vi "_memcpy.vi"(0 "MDPtr DVR":refnum<data-value>, 1 "Copy Count":i32, 5 "error in (no error)":errorcluster, 7 "Memory":string, 9 "String Attribute":string, 12 "Data Type":T1) -> (4 "MDPtr DVR(dup)":refnum<data-value>, 6 "error out":errorcluster)   [LabVIEW 2017, in "MDPtr.lvlib"]
uses:
  MDPtr.lvlib
  MDPtr TypeDef/MDPtr DataFrame-Memory.ctl
  MDPtr TypeDef/MDPtr DataFrame-Common.ctl
  <vilib>/Utility/Data Type/Type Definitions/Data Type.ctl
  _MDPtr Build Error Cluster.vi
  <vilib>/Utility/Data Type/NI_Data Type.lvlib
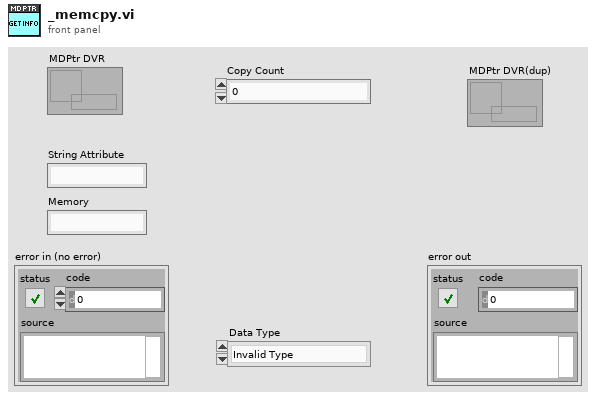
[diagram p1: front panel]
types:
  T1 = typedef "NI_Data Type.lvlib/Data Type.ctl" = enum8{"Invalid Type", "Void", "I8", "I16", "I32", "I64", "U8", "U16", "U32", "U64", "Single Float", "Double Float", "Extended Float", "Single Complex", "Double Complex", "Extended Complex", "Enum U8", "Enum U16", "Enum U32", "Enum U64", "Single Float With Unit", "Double Float With Unit", "Extended Float With Unit", "Single Complex with Unit", "Double Complex with Unit", "Extended Complex with Unit", "Boolean", "String", "Path", "Picture", "Tag", "Array", "Cluster", "Variant", "LV Variant", "Waveform", "Timestamp", "Digital Waveform", "Digital Data", "ExpressData", "Refnum", "External Data", "VI", "Poly VI", "LabVIEW Class Instance", "Fixed Point"}
  T2 = typedef "MDPtr.lvlib/MDPtr DataFrame-Memory.ctl" = cluster{"Common":T3, "DVR":refnum<data-value>}
  T3 = typedef "MDPtr.lvlib/MDPtr DataFrame-Common.ctl" = cluster{"Data Type":T1, "Copy Count":i32, "String Attribute":string, "Cache Length":i32, "Data Length":i32}
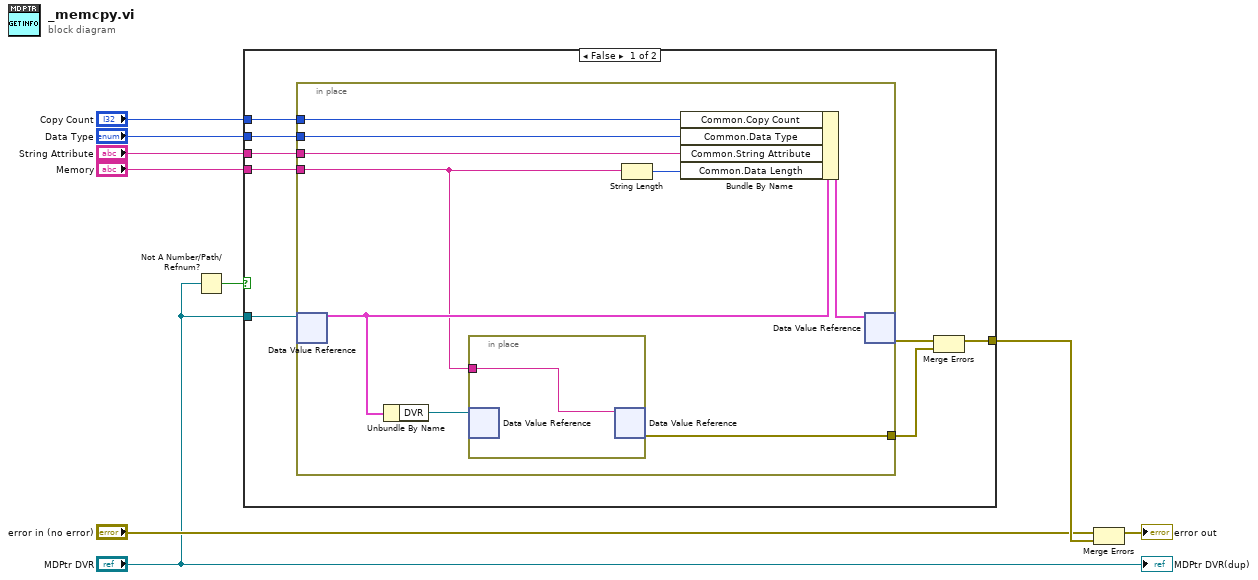
[diagram p0: block diagram]
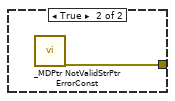
[diagram p2: hidden frame]
diagram:
  n1 = Not A Number/Path/Refnum?(number/path/refnum="MDPtr DVR") -> (NaN/Path/Refnum?=w5:bool)
  n2 = case shown="False" w5 {
    tunnel: [w11 w28] -> w9
    tunnel: "MDPtr DVR" -> [w16 _]
    tunnel: "Copy Count" -> [w15 _]
    tunnel: "Data Type" -> [w14 _]
    tunnel: "String Attribute" -> [w13 _]
    tunnel: "Memory" -> [w12 _]
    frame False {
      n3 = in-place {
        in-place-border: w15 -> [w25]
        in-place-border: w14 -> [w24]
        in-place-border: w13 -> [w23]
        in-place-border: w12 -> [w18]
        in-place-border: [w20] -> w10
        n4 = in-place-dvr #1(w16) -> (w22:T2)  [unwired: 1 out]
        n5 = Unbundle By Name(w22) -> ("DVR"=w21:refnum<data-value>)
        n6 = in-place {
          in-place-border: w18 -> [w27]
          n7 = in-place-dvr #2(w21) -> ()  [unwired: 2 out]
          n8 = in-place-dvr #2(w27) -> (w20:errorcluster)  [unwired: 1 out]
        }
        n9 = String Length(string=w18) -> (length=w19:i32)
        n10 = Bundle By Name(cluster=w22, "Common.Copy Count"=w25, "Common.Data Type"=w24, "Common.String Attribute"=w23, "Common.Data Length"=w19) -> (w26:T2)
        n11 = in-place-dvr #1(w26) -> (w17:errorcluster)  [unwired: 1 out]
      }
      n12 = Merge Errors(w17, w10) -> (w11:errorcluster)
    }
    frame True {
      n13 = call "_MDPtr NotValidStrPtr ErrorConst.vi"() -> ("error out"=w28:errorcluster)  [unwired: 19 in]
    }
  }
  n14 = Merge Errors("error in (no error)", w9) -> (→"error out":errorcluster)
  "MDPtr DVR(dup)" <- "MDPtr DVR"
